vi "Destroy.vi"(8 "Error In":errorcluster, 11 "reference in":refnum<class "G4SubTemplate_Simple_4x4x4.lvclass">) -> (0 "Error Out":errorcluster, 3 "reference out":refnum<class "G4SubTemplate_Simple_4x4x4.lvclass">)   [LabVIEW 2020, in "G4SubTemplate_Simple_4x4x4.lvclass"]
uses:
  <resource>/Framework/Providers/Open_GDS/ClassProviders/Provider_EndevoGOOP400/Templates/G4SubTemplate_Simple_4x4x4/G4SubTemplate_Simple_4x4x4.lvclass
  <resource>/Framework/Providers/Open_GDS/ClassProviders/Provider_EndevoGOOP400/Templates/G4BaseTemplate_Simple_4x4x4/G4BaseTemplate_Simple_4x4x4.lvclass
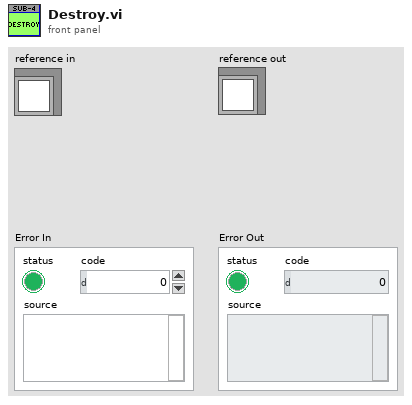
[diagram p1: front panel]
types:
  T1 = typedef "G4SubTemplate_Simple_4x4x4.lvclass/ObjectAttributes.ctl" = cluster{"Attribute1":dbl}
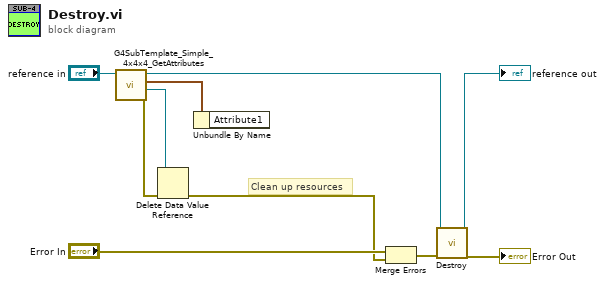
[diagram p0: block diagram]
diagram:
  # "Clean up resources"
  n1 = call <resource>:"G4SubTemplate_Simple_4x4x4_GetAttributes.vi"("reference in"="reference in") -> ("error out"=w8:errorcluster, "DataRef"=w5:refnum<data-value>, "Data"=w7:T1, "reference out"=w6:refnum<class "G4SubTemplate_Simple_4x4x4.lvclass">)  [unwired: 7 in]
  n2 = Delete Data Value Reference(data value reference=w5, error in=w8) -> (error out=w3:errorcluster)  [unwired: 1 out]
  n3 = Unbundle By Name(w7) -> ()  [unwired: 1 out]
  n4 = Merge Errors("Error In", w3) -> (w10:errorcluster)
  n5 = call-parent "Destroy.vi"("Error In"=w10, "reference in"=w6) -> ("Error Out"=→"Error Out":errorcluster, "reference out"=→"reference out":refnum<class "G4SubTemplate_Simple_4x4x4.lvclass">)  [unwired: 8 in]
